vi "error calculations.vi"(6 "Charge State":dbl=3.0, 7 "Error calculation":T1="sequence internal error", 8 "error in":errorcluster, 11 "cycle results dbl":dbl[][](array[numeric])) -> (0 "error out":errorcluster, 3 "array out":dbl[](array[numeric]))   [LabVIEW 2016]
doc: "calculates the error associated from the dead time for a\nset of cycles Deadtime(error)=(0.2*(Deadtime(%))^2"
uses:
  controls/error calculations.ctl
  <vilib>/Analysis/baseanly.llb/Mean (DBL).vi
  <vilib>/Analysis/NI_AALBase.lvlib
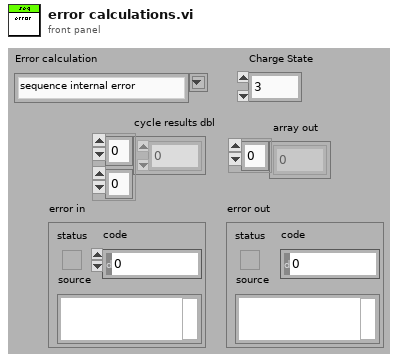
[diagram p1: front panel]
types:
  T1 = typedef "error calculations.ctl" = string
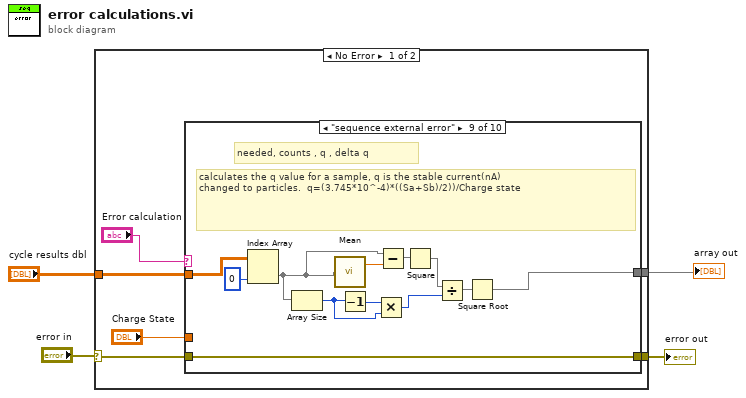
[diagram p0: block diagram]
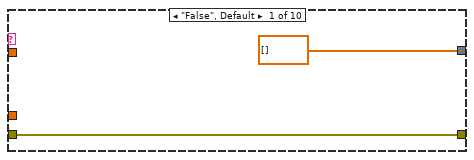
[diagram p2: hidden frame]
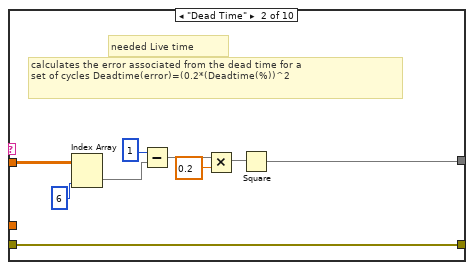
[diagram p3: hidden frame]
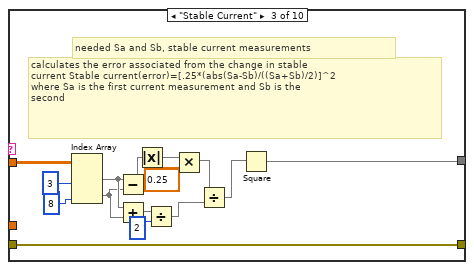
[diagram p4: hidden frame]
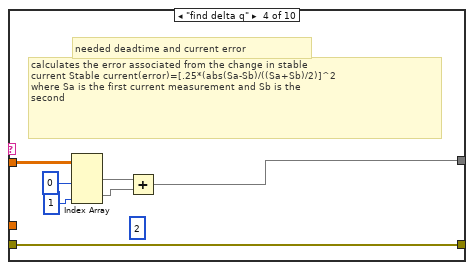
[diagram p5: hidden frame]
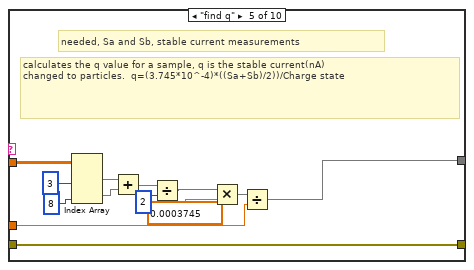
[diagram p6: hidden frame]
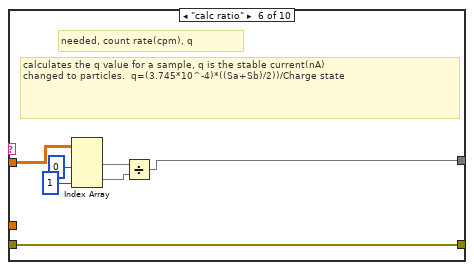
[diagram p7: hidden frame]
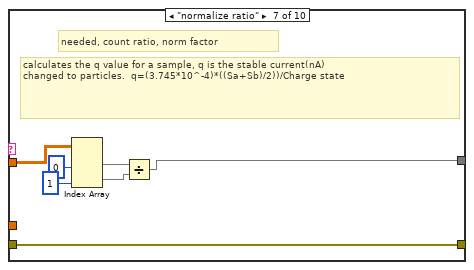
[diagram p8: hidden frame]
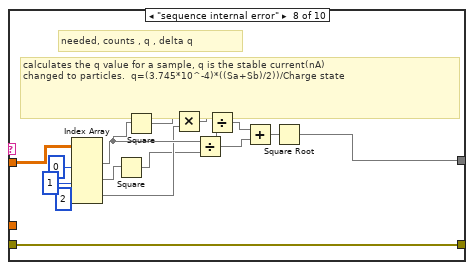
[diagram p9: hidden frame]
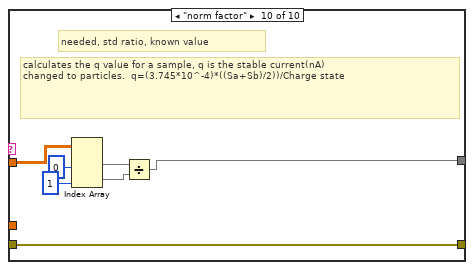
[diagram p10: hidden frame]
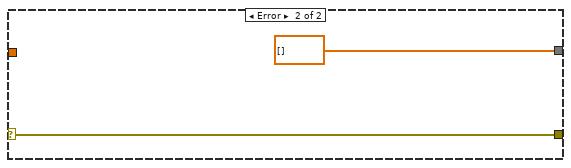
[diagram p11: hidden frame]
diagram:
  n1 = case shown="No Error" "error in" {
    selector: "error in" -> [w7 w106]
    tunnel: "cycle results dbl" -> [w10 _]
    tunnel: [w9 dbl[] []] -> w4
    tunnel: [w8 w106] -> w2
    frame No Error {
      n2 = case shown="\"sequence external error\"" "Error calculation" {
        tunnel: w10 -> [_ w15 w33 w42 w54 w62 w69 w84 w96 w103]
        tunnel: [dbl[] [] w17 w35 w37 w44 w57 w64 w71 w86 w98] -> w9
        tunnel: [w11 w16 w34 w43 w55 w63 w70 w85 w97 w104] -> w8
        tunnel: w7 -> [w11 w16 w34 w43 w55 w63 w70 w85 w97 w104]
        tunnel: "Charge State" -> [_ _ _ _ w45 _ _ _ _ _]
        frame "False", Default {
        }
        frame "Dead Time" {
          # "needed Live time"
          # "calculates the error associated from the dead time for a\nset of cycles Deadtime(error)=(0.2*(Deadtime(%))^2"
          n3 = Index Array(array=w15, index (col)=6 ("disabled index (col)")) -> (element=w13:dbl[])  [unwired: 1 in]
          n4 = Subtract(x=1 ("String"), y=w13) -> (x-y=w20:dbl[])
          n5 = Multiply(x=w20, y=0.2 ("String")) -> (x*y=w18:dbl[])
          n6 = Square(x=w18) -> (x^2=w17:dbl[])
        }
        frame "Stable Current" {
          # "needed Sa and Sb, stable current measurements"
          # "calculates the error associated from the change in stable\ncurrent Stable current(error)=[.25*(abs(Sa-Sb)/((Sa+Sb)/2)]^2\nwhere Sa is the first current measurement and Sb is the \nsecond"
          n7 = Index Array(array=w33, index (col) #1=3 ("disabled index (col)"), index (col) #2=8 ("index (col)")) -> (element #1=w30:dbl[], element #2=w29:dbl[])  [unwired: 2 in]
          n8 = Subtract(x=w30, y=w29) -> (x-y=w23:dbl[])
          n9 = Add(x=w30, y=w29) -> (x+y=w28:dbl[])
          n10 = Absolute Value(x=w23) -> (abs(x)=w22:dbl[])
          n11 = Divide(x=w28, y=2 ("String")) -> (x/y=w26:dbl[])
          n12 = Multiply(x=w22, y=0.25 ("String")) -> (x*y=w25:dbl[])
          n13 = Divide(x=w25, y=w26) -> (x/y=w24:dbl[])
          n14 = Square(x=w24) -> (x^2=w35:dbl[])
        }
        frame "find delta q" {
          (unwired) 2 ("String")
          # "needed deadtime and current error"
          # "calculates the error associated from the change in stable\ncurrent Stable current(error)=[.25*(abs(Sa-Sb)/((Sa+Sb)/2)]^2\nwhere Sa is the first current measurement and Sb is the \nsecond"
          n15 = Index Array(array=w42, index (col) #1=0 ("disabled index (col)"), index (col) #2=1 ("index (col)")) -> (element #1=w39:dbl[], element #2=w38:dbl[])  [unwired: 2 in]
          n16 = Add(x=w39, y=w38) -> (x+y=w37:dbl[])
        }
        frame "find q" {
          # "needed, Sa and Sb, stable current measurements"
          # "calculates the q value for a sample, q is the stable current(nA)\nchanged to particles.  q=(3.745*10^-4)*((Sa+Sb)/2))/Charge state"
          n17 = Index Array(array=w54, index (col) #1=3 ("disabled index (col)"), index (col) #2=8 ("index (col)")) -> (element #1=w51:dbl[], element #2=w50:dbl[])  [unwired: 2 in]
          n18 = Add(x=w51, y=w50) -> (x+y=w49:dbl[])
          n19 = Divide(x=w49, y=2 ("String")) -> (x/y=w47:dbl[])
          n20 = Multiply(x=w47, y=0.0003745 ("String")) -> (x*y=w46:dbl[])
          n21 = Divide(x=w46, y=w45) -> (x/y=w44:dbl[])
        }
        frame "calc ratio" {
          # "needed, count rate(cpm), q"
          # "calculates the q value for a sample, q is the stable current(nA)\nchanged to particles.  q=(3.745*10^-4)*((Sa+Sb)/2))/Charge state"
          n22 = Index Array(array=w62, index (col) #1=0 ("disabled index (col)"), index (col) #2=1 ("disabled index (col)")) -> (element #1=w58:dbl[], element #2=w59:dbl[])  [unwired: 2 in]
          n23 = Divide(x=w58, y=w59) -> (x/y=w57:dbl[])
        }
        frame "normalize ratio" {
          # "needed, count ratio, norm factor"
          # "calculates the q value for a sample, q is the stable current(nA)\nchanged to particles.  q=(3.745*10^-4)*((Sa+Sb)/2))/Charge state"
          n24 = Index Array(array=w69, index (col) #1=0 ("disabled index (col)"), index (col) #2=1 ("disabled index (col)")) -> (element #1=w65:dbl[], element #2=w66:dbl[])  [unwired: 2 in]
          n25 = Divide(x=w65, y=w66) -> (x/y=w64:dbl[])
        }
        frame "sequence internal error" {
          # "needed, counts , q , delta q"
          # "calculates the q value for a sample, q is the stable current(nA)\nchanged to particles.  q=(3.745*10^-4)*((Sa+Sb)/2))/Charge state"
          n26 = Index Array(array=w84, index (col) #1=0 ("disabled index (col)"), index (col) #2=1 ("disabled index (col)"), index (col) #3=2 ("index (col)")) -> (element #1=w79:dbl[], element #2=w80:dbl[], element #3=w76:dbl[])  [unwired: 3 in]
          n27 = Square(x=w80) -> (x^2=w74:dbl[])
          n28 = Square(x=w79) -> (x^2=w77:dbl[])
          n29 = Multiply(x=w77, y=w76) -> (x*y=w75:dbl[])
          n30 = Divide(x=w79, y=w74) -> (x/y=w78:dbl[])
          n31 = Divide(x=w75, y=w74) -> (x/y=w73:dbl[])
          n32 = Add(x=w73, y=w78) -> (x+y=w72:dbl[])
          n33 = Square Root(x=w72) -> (sqrt(x)=w71:dbl[])
        }
        frame "sequence external error" {
          # "needed, counts , q , delta q"
          # "calculates the q value for a sample, q is the stable current(nA)\nchanged to particles.  q=(3.745*10^-4)*((Sa+Sb)/2))/Charge state"
          n34 = Index Array(array=w96, index (col)=0 ("disabled index (col)")) -> (element=w93:dbl[])  [unwired: 1 in]
          n35 = Array Size(array=w93) -> (size(s)=w90:i32)
          n36 = call-poly <vilib>:"Mean.vi"("X"=w93) -> ("mean"=w94:dbl)  [unwired: 1 out]
          n37 = Decrement(x=w90) -> (x-1=w91:i32)
          n38 = Multiply(x=w91, y=w90) -> (x*y=w89:i32)
          n39 = Subtract(x=w93, y=w94) -> (x-y=w92:dbl[])
          n40 = Square(x=w92) -> (x^2=w88:dbl[])
          n41 = Divide(x=w88, y=w89) -> (x/y=w87:dbl[])
          n42 = Square Root(x=w87) -> (sqrt(x)=w86:dbl[])
        }
        frame "norm factor" {
          # "needed, std ratio, known value"
          # "calculates the q value for a sample, q is the stable current(nA)\nchanged to particles.  q=(3.745*10^-4)*((Sa+Sb)/2))/Charge state"
          n43 = Index Array(array=w103, index (col) #1=0 ("disabled index (col)"), index (col) #2=1 ("disabled index (col)")) -> (element #1=w99:dbl[], element #2=w100:dbl[])  [unwired: 2 in]
          n44 = Divide(x=w99, y=w100) -> (x/y=w98:dbl[])
        }
      }
    }
    frame Error {
    }
  }
  "array out" <- w4
  "error out" <- w2
